vi "Synthesize.vi"(0 "Noise in":refnum<class "Noise.lvclass">, 5 "Fs (Hz)":dbl, 7 "Npts":i32, 9 "Repetition":i32, 11 "error in (no error)":errorcluster) -> (4 "Noise out":refnum<class "Noise.lvclass">, 8 "Array":dbl[](array[numeric]), 15 "error out":errorcluster)   [LabVIEW 2020, in "Noise.lvclass"]
uses:
  Noise.lvclass
  Noise.lvclass/Noise.ctl
  <vilib>/Analysis/NI_AALBase.lvlib
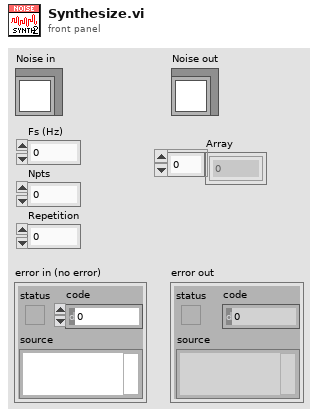
[diagram p1: front panel]
types:
  T1 = enum16{"Clear", "Set data", "Reset index", "Get data"}
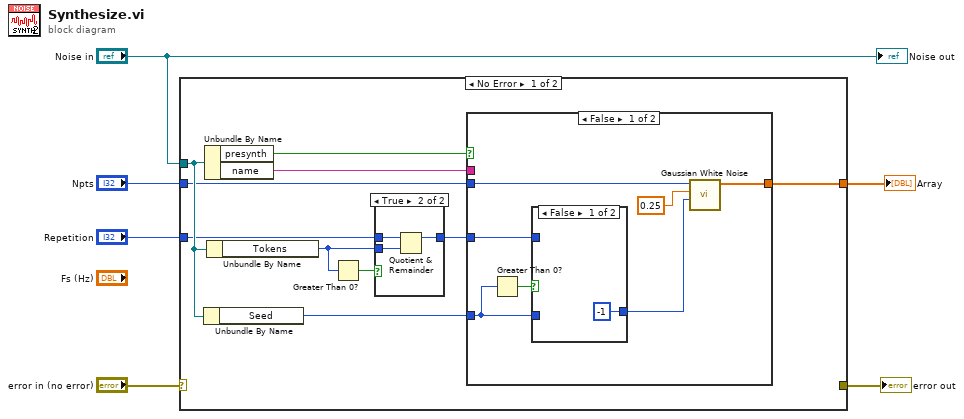
[diagram p0: block diagram]
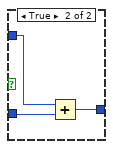
[diagram p2: hidden frame]
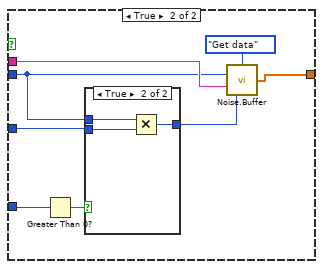
[diagram p3: hidden frame]
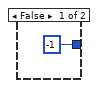
[diagram p4: hidden frame]
diagram:
  n1 = case shown="No Error" "error in (no error)" {
    selector: "error in (no error)" -> [_ w44]
    tunnel: "Noise in" -> [w15 _]
    tunnel: [_ w44] -> w4
    tunnel: "Repetition" -> [w12 _]
    tunnel: "Npts" -> [w9 _]
    tunnel: [w8 _] -> w1
    frame No Error {
      n2 = Unbundle By Name(w15) -> ("Seed"=w10:i32)
      n3 = Unbundle By Name(w15) -> ("presynth"=w16:bool, "name"=w7:string)
      n4 = Unbundle By Name(w15) -> ("Tokens"=w13:i32)
      n5 = Greater Than 0?(x=w13) -> (x > 0?=w14:bool)
      n6 = case shown="True" w14 {
        tunnel: w13 -> [_ w43]
        tunnel: [w40 w42] -> w11
        tunnel: w12 -> [w40 w41]
        frame False {
        }
        frame True {
          n7 = Quotient & Remainder(x=w41, y=w43) -> (x-y*floor(x/y)=w42:i32)  [unwired: 1 out]
        }
      }
      n8 = case shown="False" w16 {
        tunnel: w11 -> [w21 w31]
        tunnel: w10 -> [w22 w30]
        tunnel: w9 -> [w20 w28]
        tunnel: [w17 w33] -> w8
        tunnel: w7 -> [_ w34]
        frame False {
          n9 = Greater Than 0?(x=w22) -> (x > 0?=w23:bool)
          n10 = case shown="False" w23 {
            tunnel: w22 -> [_ w27]
            tunnel: w21 -> [_ w26]
            tunnel: [-1 w25] -> w19
            frame False {
            }
            frame True {
              n11 = Add(x=w26, y=w27) -> (x+y=w25:i32)
            }
          }
          n12 = call <vilib>:"Gaussian White Noise.vi"("seed"=w19, "standard deviation"=0.25, "samples"=w20) -> ("Gaussian noise pattern"=w17:dbl[])  [unwired: 7 in, 1 out]
        }
        frame True {
          n13 = Greater Than 0?(x=w30) -> (x > 0?=w32:bool)
          n14 = case shown="True" w32 {
            tunnel: w31 -> [_ w38]
            tunnel: w28 -> [_ w39]
            tunnel: [-1 w37] -> w29
            frame False {
            }
            frame True {
              n15 = Multiply(x=w39, y=w38) -> (x*y=w37:i32)
            }
          }
          n16 = call "Noise.Buffer.vi"("Action"=T1."Get data", "Npts"=w28, "Name"=w34, "offset"=w29) -> ("Data Out"=w33:dbl[])  [unwired: 10 in, 1 out]
        }
      }
    }
    frame Error {
    }
  }
  "error out" <- w4
  "Array" <- w1
  "Noise out" <- "Noise in"
